vi "testConverDatatype2.vi"(11 "s in":string) -> (3 "s out":string)   [LabVIEW 2011]
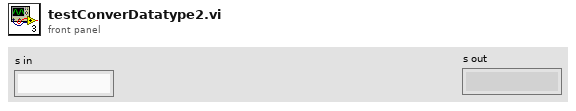
[diagram p1: front panel]
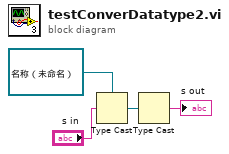
[diagram p0: block diagram]
diagram:
  n1 = Type Cast(type=refnum<queue> refnum ("队列输出"), x="s in") -> (*(type *) &x=w2:refnum<queue>)
  n2 = Type Cast(x=w2) -> (*(type *) &x=→"s out":string)  [unwired: 1 in]
